vi "return_to_origin.vi"(8 "error in (no error)":errorcluster, 11 "StageDL090409Scaffold in":refnum<class "StageDL090409Scaffold.lvclass">) -> (0 "error out":errorcluster, 3 "StageDL090409Scaffold out":refnum<class "StageDL090409Scaffold.lvclass">)   [LabVIEW 2010, in "StageDL090409Scaffold.lvclass"]
uses:
  StageDL090409Scaffold.lvclass
  GenericStage/GenericStage/translation_mode_enum.ctl
  StageDL090409Scaffold.lvclass/StageDL090409Scaffold.ctl
  GenericStage/GenericStage/GenericStage.lvclass
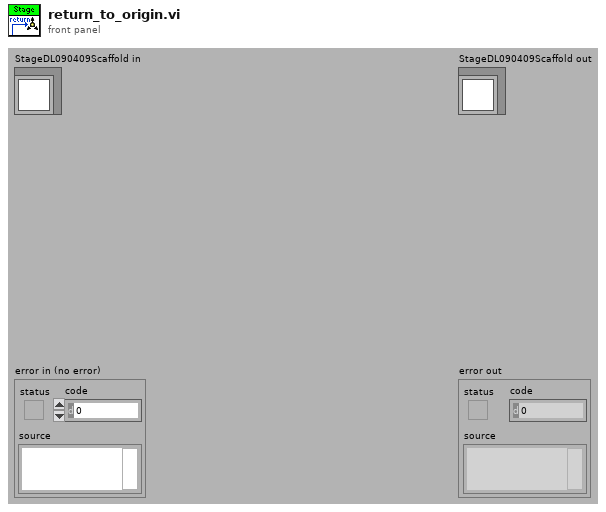
[diagram p1: front panel]
types:
  T1 = typedef "GenericStage.lvclass/translation_mode_enum.ctl" = enum16{"DON'T MOVE", "relative", "absolute"}
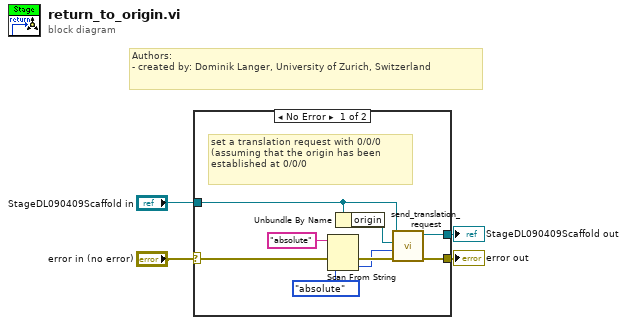
[diagram p0: block diagram]
diagram:
  # "Authors: \n- created by: Dominik Langer, University of Zurich, Switzerland"
  n1 = case shown="No Error" "error in (no error)" {
    selector: "error in (no error)" -> [w9 w15]
    tunnel: [w13 w15] -> w3
    tunnel: [w10 w14] -> w1
    tunnel: "StageDL090409Scaffold in" -> [w11 w14]
    frame No Error {
      # "set a translation request with 0/0/0 (assuming that the origin has been established at 0/0/0"
      n2 = Scan From String(input string="absolute", error in=w9, default 1=translation_mode_enum."absolute" ("translation mode")) -> (error out=w8:errorcluster, output 1=w5:T1)  [unwired: 2 in, 2 out]
      n3 = Unbundle By Name(w11) -> ("origin"=w12:refnum<class "SpaceVector.lvclass">)
      n4 = call-dynamic "send_translation_request.vi"("error in (no error)"=w8, "translation mode"=w5, "translation vector"=w12, "GenericStage in"=w11) -> ("error out"=w13:errorcluster, "GenericStage out"=w10:refnum<class "StageDL090409Scaffold.lvclass">)  [unwired: 6 in]
    }
    frame Error {
    }
  }
  "error out" <- w3
  "StageDL090409Scaffold out" <- w1
